vi "Get Alias Mappings from Channel ID.vi"(8 "error in (no error)":errorcluster, 11 "Routing Channel Ref in":T1 format="%.0x") -> (0 "error out":errorcluster, 2 "Alias Mappings":T2[](array[typedef]), 3 "Routing Channel Ref out":T1 format="%.0x")   [LabVIEW 2017, in "Routing and Faulting System Explorer.lvlib"]
uses:
  Routing and Faulting System Explorer.lvlib
  Shared/Alias Mapping.ctl
  <vilib>/NI Veristand/Custom Device API/Custom Device Item Ref.ctl
  Scripting/Routing and Faulting Scripting.lvlib
  <vilib>/NI VeriStand/Custom Device API/Custom Device API.lvlib
  Shared/Routing and Faulting Shared.lvlib
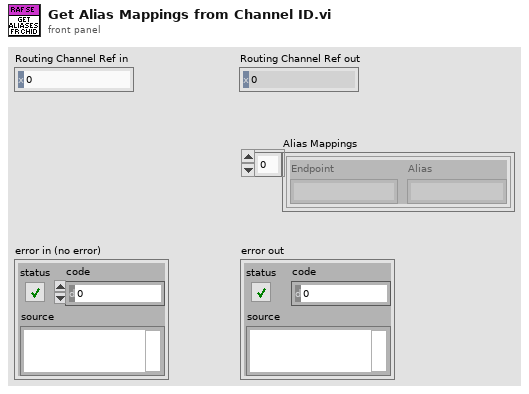
[diagram p1: front panel]
types:
  T1 = typedef "Custom Device API.lvlib/Custom Device Item Ref.ctl" = u64
  T2 = typedef "Routing and Faulting Shared.lvlib/Alias Mapping.ctl" = cluster{"Endpoint":string, "Alias":string}
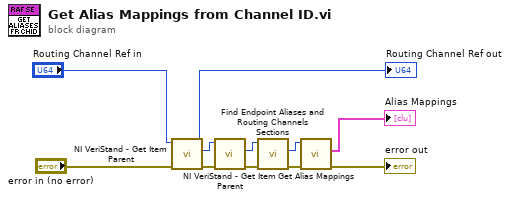
[diagram p0: block diagram]
diagram:
  n1 = call <vilib>:"NI VeriStand - Get Item Parent.vi"("error in (no error)"="error in (no error)", "Item Ref in"="Routing Channel Ref in") -> ("error out"=w7:errorcluster, "Parent Ref"=w8:T1, "Item Ref out"=→"Routing Channel Ref out":T1)  [unwired: 6 in, 1 out]
  n2 = call <vilib>:"NI VeriStand - Get Item Parent.vi"("error in (no error)"=w7, "Item Ref in"=w8) -> ("error out"=w10:errorcluster, "Parent Ref"=w9:T1)  [unwired: 6 in, 2 out]
  n3 = call "Find Endpoint Aliases and Routing Channels Sections.vi"("error in (no error)"=w10, "Routing and Faulting Custom Device Ref in"=w9) -> ("error out"=w5:errorcluster, "Endpoint Aliases Ref"=w4:T1)  [unwired: 6 in, 2 out]
  n4 = call "Get Alias Mappings.vi"("error in (no error)"=w5, "Endpoint Aliases Ref in"=w4) -> ("error out"=→"error out":errorcluster, "Alias Mappings"=→"Alias Mappings":T2[])  [unwired: 7 in, 1 out]
